vi "FindMatchEqualizationPoints.vi"(11 "RawSchedule":string[][](array[string])) -> (2 "Array 2":string[][](array[string]), 3 "Array":i32[](array[numeric]))   [LabVIEW 2013]
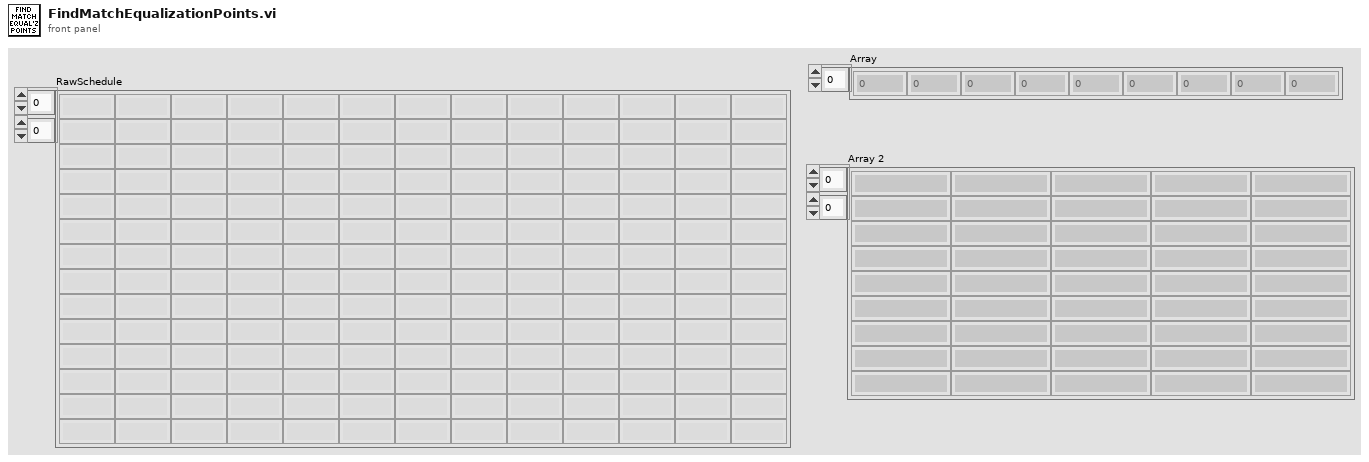
[diagram p1: front panel]
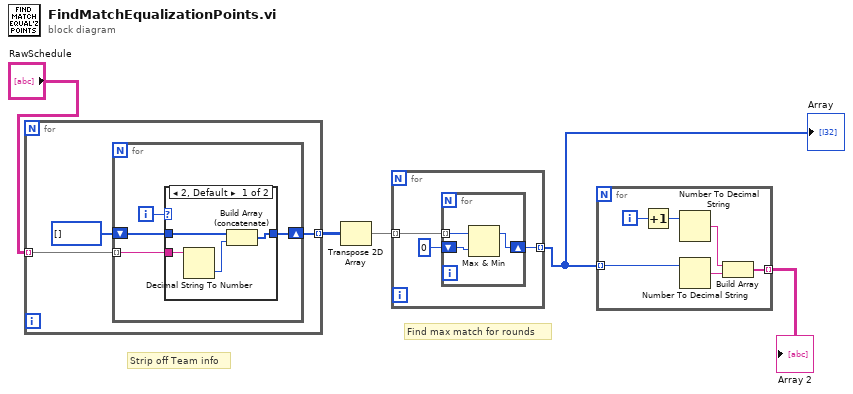
[diagram p0: block diagram]
diagram:
  # "Find max match for rounds"
  # "Strip off Team info"
  n1 = for {
    tunnel: "RawSchedule" -> [w8] mode=indexing
    tunnel: [w6] -> w2 mode=indexing
    n2 = for {
      tunnel: w8 -> [w11] mode=indexing
      shift-right: [w9] -> w6
      shift-left: i32[] [] -> [w10]
      i -> [w12]
      n3 = case shown="2, Default" w12 {
        tunnel: w11 -> [w16 _]
        tunnel: w10 -> [w15 w17]
        tunnel: [w13 w17] -> w9
        frame 2, Default {
          n4 = Decimal String To Number(string=w16) -> (number=w14:i32)  [unwired: 2 in, 1 out]
          n5 = Build Array (concatenate)(w15, w14) -> (w13:i32[])
        }
        frame 0, 1 {
        }
      }
    }
  }
  n6 = Transpose 2D Array(2D array=w2) -> (transposed array=w3:i32[][])
  n7 = for {
    tunnel: w3 -> [w19] mode=indexing
    tunnel: [w18] -> w5 mode=indexing
    n8 = for {
      shift-right: [w21] -> w18
      shift-left: 0 -> [w22]
      tunnel: w19 -> [w23] mode=indexing
      n9 = Max & Min(x=w23, y=w22) -> (max(x,y)=w21:i32)  [unwired: 1 out]
    }
  }
  "Array" <- w5
  n10 = for {
    tunnel: [w25] -> w4 mode=indexing
    tunnel: w5 -> [w24] mode=indexing
    i -> [w28]
    n11 = Increment(x=w28) -> (x+1=w29:i32)
    n12 = Number To Decimal String(number=w29) -> (decimal integer string=w27:string)  [unwired: 1 in]
    n13 = Number To Decimal String(number=w24) -> (decimal integer string=w26:string)  [unwired: 1 in]
    n14 = Build Array(w27, w26) -> (w25:string[])
  }
  "Array 2" <- w4
